vi "autohideHScrollbar.vi"(8 "error in (no error)":errorcluster, 10 "Table in":refnum<vi>, 11 "State":T1={"logTable"=refnum, "max items"=500, "displaydata"=[], "data"=[], "Auto Scroll"=TRUE, "current item"=500, "col headers"=[], "Add to Top"=TRUE, "Auto resize"=TRUE, "col size"=[], "filters"=[], "color cells"=[]}) -> (0 "error out":errorcluster, 2 "Table out":refnum<vi>, 3 "State (dup)":T1={"logTable"=refnum, "max items"=500, "displaydata"=[], "data"=[], "Auto Scroll"=TRUE, "current item"=500, "col headers"=[], "Add to Top"=TRUE, "Auto resize"=TRUE, "col size"=[], "filters"=[], "color cells"=[]})   [LabVIEW 2017, in "UI-DisplayTable(dev).xctl"]
uses:
  UI-DisplayTable(dev).xctl
  State.ctl
  DEF-Filter.ctl
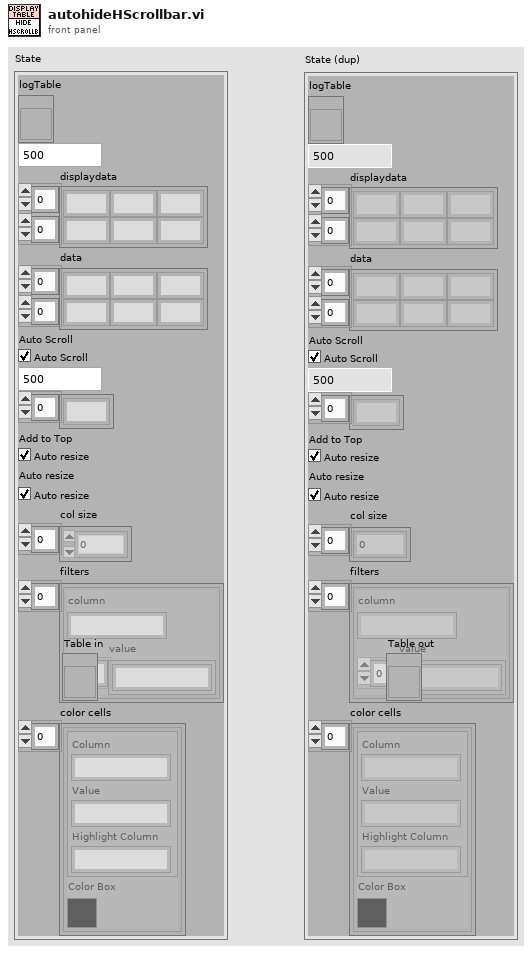
[diagram p1: front panel]
types:
  T1 = typedef "UI-DisplayTable(dev).xctl/State.ctl" = cluster{"logTable":refnum<vi>, "max items":i32, "displaydata":string[][], "data":string[][], "Auto Scroll":bool, "current item":i32, "col headers":string[], "Add to Top":bool, "Auto resize":bool, "col size":i32[], "filters":T2[], "color cells":cluster{"color cell":cluster{"Column":string, "Value":string, "Highlight Column":string}, "Color Box":u32}[]}
  T2 = typedef "UI-DisplayTable(dev).xctl/DEF-Filter.ctl" = cluster{"column":string, "value":string[]}
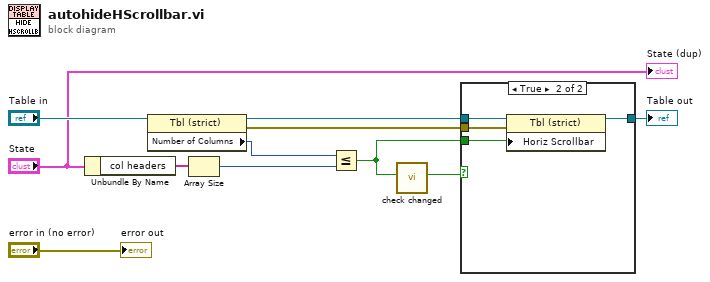
[diagram p0: block diagram]
diagram:
  n1 = Unbundle By Name("State") -> ("col headers"=w7:string[])
  n2 = property class="Tbl (strict)"(reference="Table in") -> (reference out=w6:refnum<vi>, error out=w5:errorcluster, "Number of Columns"=w4:u32)  [unwired: 1 in]
  n3 = Array Size(array=w7) -> (size(s)=w3:i32)
  n4 = Less Or Equal?(x=w4, y=w3) -> (x <= y?=w2:bool)
  n5 = call "check changed.vi"("data"=w2) -> ("changed?"=w1:bool)  [unwired: 9 in, 1 out]
  n6 = case shown="True" w1 {
    tunnel: [w12 w16] -> w9
    tunnel: w6 -> [w12 w15]
    tunnel: w5 -> [_ w14]
    tunnel: w2 -> [_ w13]
    frame False {
    }
    frame True {
      n7 = property class="Tbl (strict)"(reference=w15, error in=w14, "Horiz Scrollbar"=w13) -> (reference out=w16:refnum<vi>)  [unwired: 1 out]
    }
  }
  "Table out" <- w9
  "error out" <- "error in (no error)"
  "State (dup)" <- "State"
